vi "4110_Global.vi"() -> ()   [LabVIEW 2018, in "NI PXI-4110 Programmable Power Supply Custom Device.lvlib"]
uses:
  NI PXI-4110 Programmable Power Supply Custom Device.lvlib
panel:
  in  "Current Chan RTM GUID":string="a75eced0-4074-47c0-908c-c3062bedfbe5"
  in  "Volt Chan RTM GUID":string="a75eced0-4074-47c0-908c-c3062bedfbe5"
  in  "Hardware Type":string="Hardware Type"
  in  "Power Supply":string="Power Supply"
  in  "Initial C Value":string="Initial C Value"
  in  "Channel Name":string="Channel #"
  in  "Channel Page GUID":string="a75eced0-4074-47c0-908c-c3062bedfbe5"
  in  "Voltage Limit":string="Voltage Limit"
  in  "Current Limit":string="Current Limit"
  in  "Initial V Value":string="Initial V Value"
  in  "Sense":string="Sense"
  in  "IO Type":string="IO Type"
  in  "Channel #":string="Channel #"
  in  "Device Name":string="Device Name"
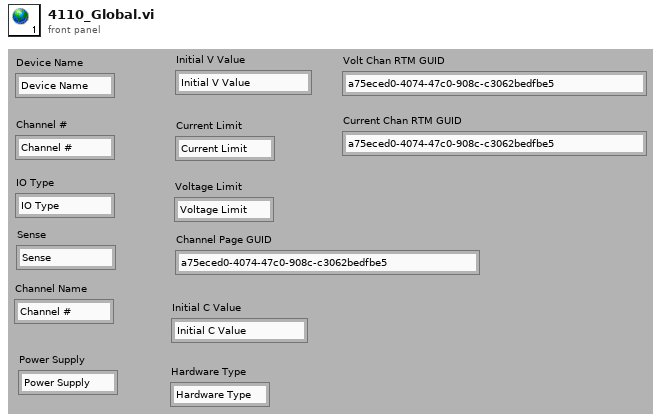
[diagram p1: front panel]
diagram:
